vi "Current Value.vi"(8 "error in (no error)":errorcluster, 11 "Channel in":refnum<class "Channel DBL.lvclass">) -> (0 "error out":errorcluster, 1 "Timestamp":dbl, 2 "Scaled":dbl, 3 "Channel out":refnum<class "Channel DBL.lvclass">, 4 "Raw":dbl)   [LabVIEW 2020, in "Vecto.lvlib" / "Channel DBL.lvclass"]
uses:
  Channel DBL.lvclass
  Channel DBL.lvclass/Channel DBL.ctl
  Group DBL/Group DBL.lvclass
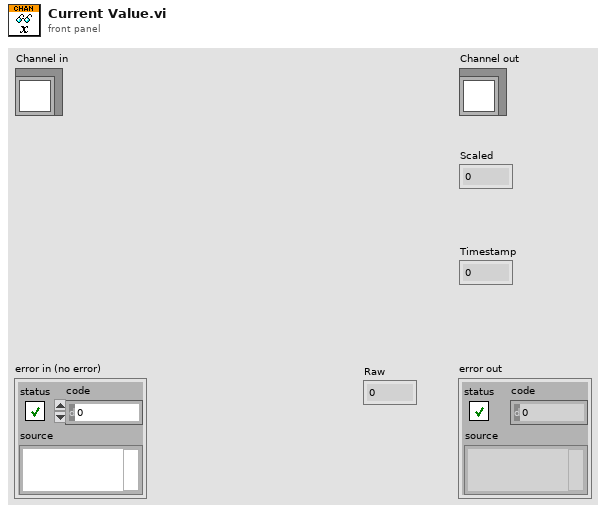
[diagram p1: front panel]
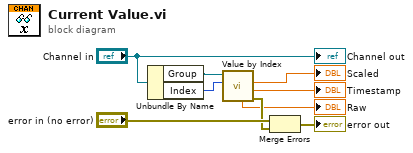
[diagram p0: block diagram]
diagram:
  n1 = Unbundle By Name("Channel in") -> ("Group"=w6:refnum<class "Group DBL.lvclass">, "Index"=w5:i32)
  n2 = call "Value by Index.vi"("Index"=w5, "Group in"=w6) -> ("error out"=w4:errorcluster, "Timestamp"=→"Timestamp":dbl, "Scaled"=→"Scaled":dbl, "Raw"=→"Raw":dbl)  [unwired: 5 in, 1 out]
  n3 = Merge Errors("error in (no error)", w4) -> (→"error out":errorcluster)
  "Channel out" <- "Channel in"
